vi "guid.vi"() -> (0 "error out":errorcluster, 3 "GUID":string)   [LabVIEW 2019]
doc: "Generate GUID"
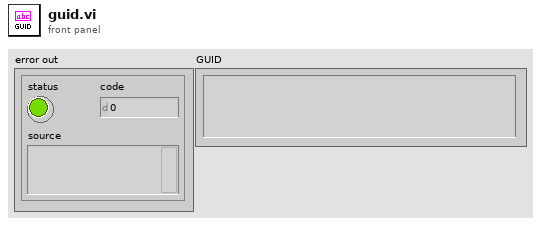
[diagram p1: front panel]
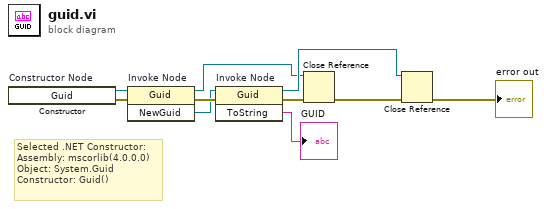
[diagram p0: block diagram]
diagram:
  # "Selected .NET Constructor:\nAssembly: mscorlib(4.0.0.0)\nObject: System.Guid\nConstructor: Guid()"
  n1 = constructor on="Constructor Node" class="System.Guid"() -> (reference out=w1:refnum<k24>, error out=w2:errorcluster)  [unwired: 3 in, 1 out]
  n2 = invoke on="Invoke Node" class="Guid" method="NewGuid"(reference=w1, error in=w2) -> (reference out=w7:refnum<k24>, error out=w4:errorcluster, "NewGuid"=w3:refnum<k24>)  [unwired: 1 in]
  n3 = invoke on="Invoke Node" class="Guid" method="ToString"(reference=w3, error in=w4) -> (reference out=w8:refnum<k24>, error out=w5:errorcluster, "ToString"=→"GUID":string)  [unwired: 1 in]
  n4 = Close Reference(reference=w7, error in (no error)=w5) -> (error out=w6:errorcluster)
  n5 = Close Reference(reference=w8, error in (no error)=w6) -> (error out=→"error out":errorcluster)
